vi "instrumentProperties_channels.vi"(8 "error in (no error)":errorcluster, 11 "OSA300 in":refnum<class "OSA300.lvclass">) -> (0 "error out":errorcluster, 1 "channel properties":T2[](array[typedef]), 2 "channels nr":i32, 3 "OSA300 out":refnum<class "OSA300.lvclass">, 4 "channelType_spectrum":T1, 5 "channel DUT (index)":i32)   [LabVIEW 2010, in "OSA300.lvclass"]
uses:
  OSA300.lvclass
  _misc/Thorlabs_FTS_misc.llb/channel_propertiesGen.ctl
  _misc/Thorlabs_FTS_misc.llb/detector_sort.ctl
  _misc/Thorlabs_FTS_misc.llb/channelType_spectrum.ctl
  _OSAchannel_class/OSAchannel.lvclass
  OSA20X_misc.lvlib
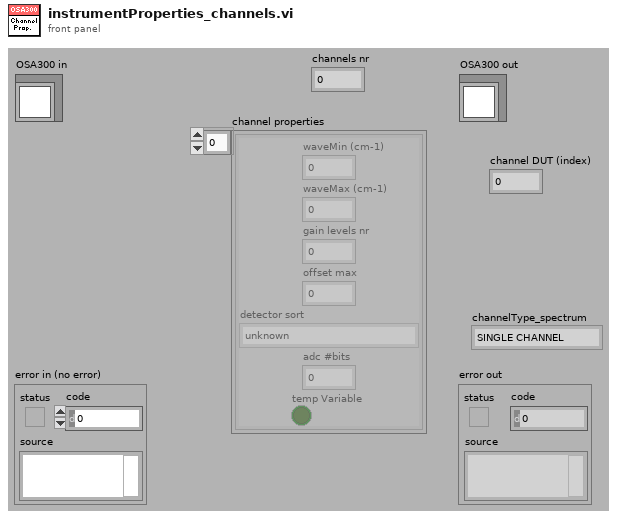
[diagram p1: front panel]
types:
  T1 = typedef "OSA20X_misc.lvlib/channelType_spectrum.ctl" = enum16{"SINGLE CHANNEL", "STICHED"}
  T2 = typedef "OSA20X_misc.lvlib/channel_propertiesGen.ctl" = cluster{"waveMin (cm-1)":sgl, "waveMax (cm-1)":sgl, "gain levels nr":u16, "offset max":u16, "detector sort":T3, "adc #bits":u16, "temp Variable":bool}
  T3 = typedef "OSA20X_misc.lvlib/detector_sort.ctl" = enum16{"unknown", "Silicon", "Silicon PIN", "Silicon MPPC", "InGaAs", "InGaAs ext low", "InGaAs ext high", "InAs", "InAsSb", "InSb", "MCT", "other", "other2", "other3"}
  T4 = typedef "OSA20X_misc.lvlib/amplifier_sort.ctl" = enum16{"amp_unknown", "amp_se_8", "amp_se_12_lg", "amp_se_12", "amp_se_16", "amp_diff_8", "amp_diff_12_lg", "amp_diff_12_ir", "amp_diff_16", "amp_other", "amp_other_2"}
  T5 = typedef "OSA20X_misc.lvlib/interferogram_smoothing.ctl" = enum16{"NONE", "BINOMIAL", "SAVITSKY_GOLAY", "FOURIER", "MOVING_AVERAGE", "GAUSSIAN"}
  T6 = typedef "OSA20X_misc.lvlib/PDTemperatureMode.ctl" = enum16{"cool: better sensitivity/noise floor", "warm: extended wl range"}
  T7 = cluster{"waveMin (cm-1)":sgl, "waveMax (cm-1)":sgl, "gainOffset_auto":bool, "gain":i32, "gain levels nr":u16, "offset":i32, "offset max":u16, "damper available":bool, "damper active":bool, "amplifier sort":T4, "detector sort":T3, "channelIdx global":u16, "spectrIdx":u16, "waveMeter on":bool, "ref gainLevels rel.":refnum<data-value>, "intfgrm_smooth_width":u16, "intfgrm_smooth_nrOfPasses":u16, "intfgrm_smooth":T5, "adc #bits":u16, "temp Variable":bool, "spectr_smooth":T5, "spectr_smooth_width":u16, "spectr_smooth_nrOfPasses":u16, "PD sensitivity mode":T6}
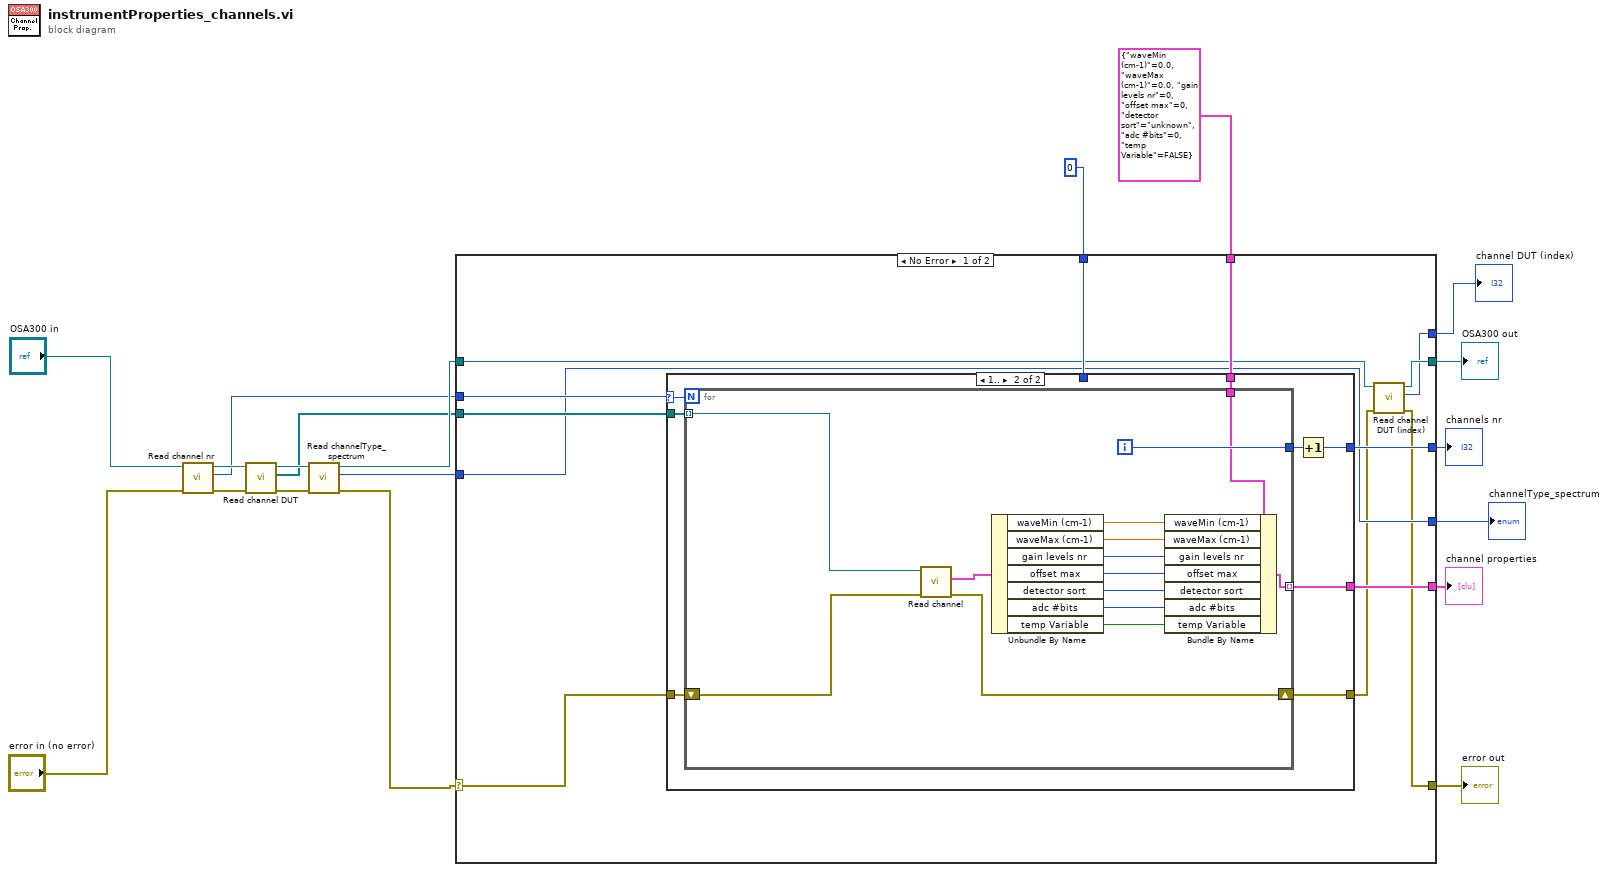
[diagram p0: block diagram]
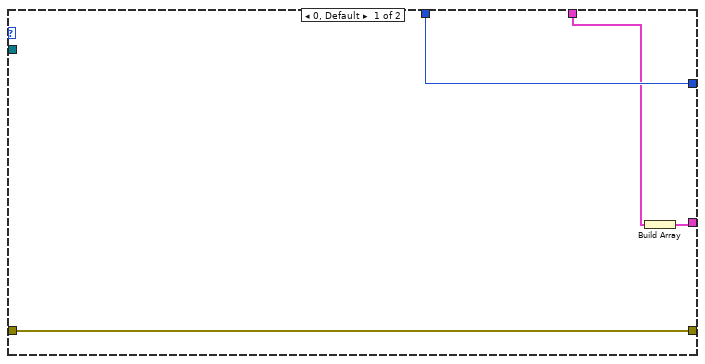
[diagram p2: hidden frame]
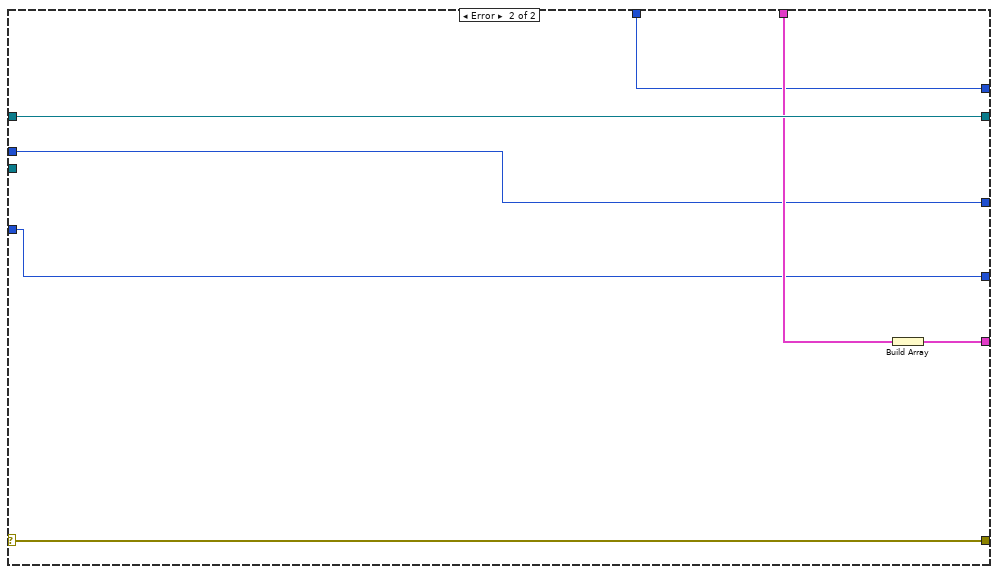
[diagram p3: hidden frame]
diagram:
  n1 = call "Read channel nr.vi"("error in (no error)"="error in (no error)", "OSA300 in"="OSA300 in") -> ("error out"=w4:errorcluster, "channel nr"=w2:i32, "OSA300 out"=w7:refnum<class "OSA300.lvclass">)  [unwired: 7 in]
  n2 = call "Read channel DUT.vi"("error in (no error)"=w4, "OSA300 in"=w7) -> ("error out"=w3:errorcluster, "channel DUT"=w1:refnum<class "OSAchannel.lvclass">[], "OSA300 out"=w6:refnum<class "OSA300.lvclass">)  [unwired: 7 in]
  n3 = call "Read channelType_spectrum.vi"("error in (no error)"=w3, "OSA300 in"=w6) -> ("error out"=w11:errorcluster, "channelType_spectrum"=w10:T1, "OSA300 out"=w9:refnum<class "OSA300.lvclass">)  [unwired: 7 in]
  n4 = case shown="No Error" w11 {
    selector: w11 -> [w32 w65]
    tunnel: [w21 w65] -> w19
    tunnel: [w23 w64] -> w18
    tunnel: w9 -> [w24 w64]
    tunnel: [w31 w60] -> w17
    tunnel: [w30 w63] -> w16
    tunnel: 0 -> [w28 w61]
    tunnel: T2 {"waveMin (cm-1)"=0.0, "waveMax (cm-1)"=0.0, "gain levels nr"=0, "offset max"=0, "detector sort"=enum."unknown", "adc #bits"=0, "temp Variable"=FALSE} -> [w29 w62]
    tunnel: [w20 w61] -> w13
    tunnel: w2 -> [w27 w60]
    tunnel: w1 -> [w26 _]
    tunnel: [w25 w59] -> w12
    tunnel: w10 -> [w25 w59]
    frame No Error {
      n5 = case shown="1.." w27 {
        selector: w27 -> [_ w42]
        tunnel: w26 -> [_ w44]
        tunnel: w32 -> [w36 w43]
        tunnel: [w35 w40] -> w31
        tunnel: [w34 w39] -> w30
        tunnel: [w36 w38] -> w22
        tunnel: w29 -> [w33 w37]
        tunnel: w28 -> [w35 _]
        frame 0, Default {
          n6 = Build Array(w33) -> (w34:T2[])
        }
        frame 1.. {
          n7 = for {
            N: w42 -> [_]
            tunnel: w44 -> [w58] mode=indexing
            shift-right: [w54] -> w38
            shift-left: w43 -> [w57]
            tunnel: [w55] -> w41
            tunnel: [w52] -> w39 mode=indexing
            tunnel: w37 -> [w53]
            i -> [w55]
            n8 = call "Read channel.vi"("error in (no error)"=w57, "OSAchannel in"=w58) -> ("error out"=w54:errorcluster, "channel"=w56:T7)  [unwired: 7 in, 1 out]
            n9 = Unbundle By Name(w56) -> ("waveMin (cm-1)"=w51:sgl, "waveMax (cm-1)"=w50:sgl, "gain levels nr"=w49:u16, "offset max"=w48:u16, "detector sort"=w47:T3, "adc #bits"=w46:u16, "temp Variable"=w45:bool)
            n10 = Bundle By Name(cluster=w53, "waveMin (cm-1)"=w51, "waveMax (cm-1)"=w50, "gain levels nr"=w49, "offset max"=w48, "detector sort"=w47, "adc #bits"=w46, "temp Variable"=w45) -> (w52:T2)
          }
          n11 = Increment(x=w41) -> (x+1=w40:i32)
        }
      }
      n12 = call "Read channel DUT (index).vi"("error in (no error)"=w22, "OSA300 in"=w24) -> ("error out"=w21:errorcluster, "channel ifrgrm (index)"=w20:i32, "OSA300 out"=w23:refnum<class "OSA300.lvclass">)  [unwired: 7 in]
    }
    frame Error {
      n13 = Build Array(w62) -> (w63:T2[])
    }
  }
  "error out" <- w19
  "OSA300 out" <- w18
  "channels nr" <- w17
  "channel properties" <- w16
  "channel DUT (index)" <- w13
  "channelType_spectrum" <- w12
